vi "OE.vi"(2 "report in":refnum<class "NI_report.lvclass">, 3 "表格数据路径：":path=path "C:/Users/shipeng/Desktop/LT Dielectric measurement", 5 "Array":string[][](array[string]), 6 "String 4":string, 7 "String":string, 8 "error in (no error)":errorcluster, 9 "String 3":string, 10 "String 2":string, 11 "Numeric":u16) -> (0 "error out":errorcluster, 1 "report out":refnum<class "NI_report.lvclass">, 4 "Array 2":string[][](array[string]))   [LabVIEW 2017]
uses:
  <vilib>/Utility/NIReport.llb/NI_report.lvclass
  <vilib>/addons/_office/excel.llb/Excel Easy Table (str).vi
  <vilib>/addons/_office/NI_ReportGenerationToolkit.lvlib
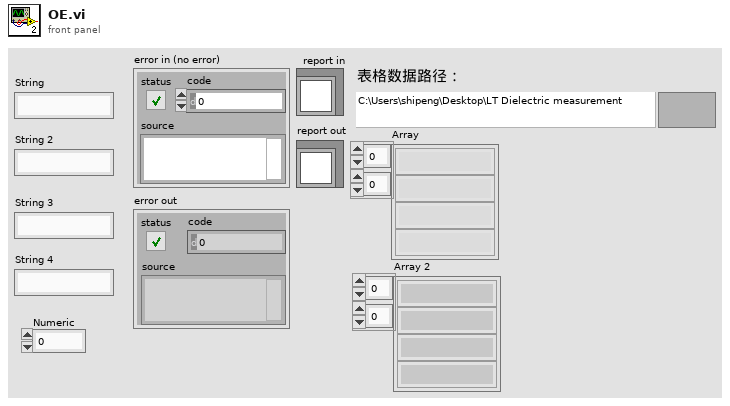
[diagram p1: front panel]
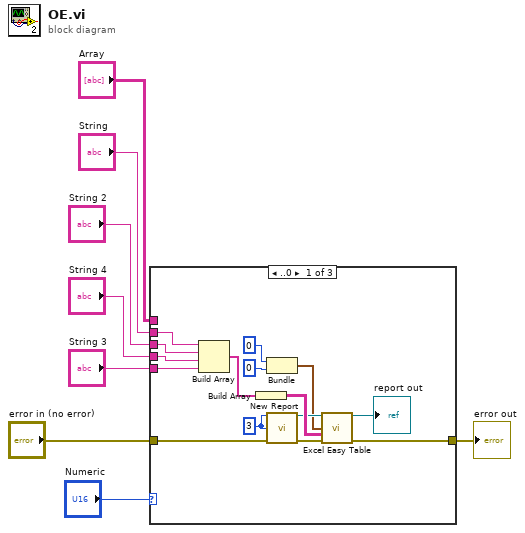
[diagram p0: block diagram]
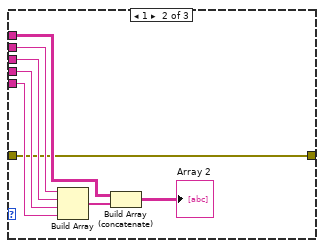
[diagram p2: hidden frame]
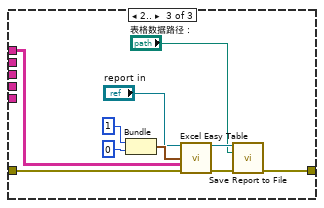
[diagram p3: hidden frame]
diagram:
  n1 = case shown="..0" "Numeric" {
    tunnel: "String 4" -> [w14 w27 _]
    tunnel: "String 3" -> [w13 w26 _]
    tunnel: "String 2" -> [w12 w28 _]
    tunnel: "String" -> [w11 w29 _]
    tunnel: "Array" -> [_ w25 w34]
    tunnel: "error in (no error)" -> [w10 w24 w32]
    tunnel: [w9 w24 w33] -> w1
    frame ..0 {
      w22 = 3
      n2 = Build Array(w11, w12, w14, w13) -> (w23:string[])
      n3 = Build Array(w23) -> (w21:string[][])
      n4 = Bundle(0, 0) -> (w19:cluster{i32, i32})  [unwired: 1 in]
      n5 = call <vilib>:"New Report.vi"("window state (normal)"=w22, "report type"=w22, "error in (no error)"=w10) -> ("report out"=w20:refnum<class "NI_report.lvclass">, "error out"=w18:errorcluster)  [unwired: 11 in]
      n6 = call-poly <vilib>:"Excel Easy Table.vi"("report in"=w20, "start (0, 0)"=w19, "text data"=w21, "error in (no error)"=w18) -> ("report out"=→"report out":refnum<class "NI_report.lvclass">, "error out"=w9:errorcluster)  [unwired: 7 in, 3 out]
    }
    frame 1 {
      n7 = Build Array(w29, w28, w27, w26) -> (w31:string[])
      n8 = Build Array (concatenate)(w25, w31) -> (→"Array 2":string[][])
    }
    frame 2.. {
      n9 = Bundle(1, 0) -> (w41:cluster{i32, i32})  [unwired: 1 in]
      n10 = call-poly <vilib>:"Excel Easy Table.vi"("report in"="report in", "start (0, 0)"=w41, "text data"=w34, "error in (no error)"=w32) -> ("report out"=w40:refnum<class "NI_report.lvclass">, "error out"=w39:errorcluster)  [unwired: 7 in, 3 out]
      n11 = call-dynamic "Save Report to File.vi"("report in"=w40, "report file path"="表格数据路径：", "error in (no error)"=w39) -> ("error out"=w33:errorcluster)  [unwired: 11 in, 1 out]
    }
  }
  "error out" <- w1
